vi "氨氮测量流程.vi"(10 "量程模式":T1, 11 "参数":T2={"站号"=1, "量程切换"=enum."AUTO", "控制命令"=enum."启动测量", "模式设置"=enum."待机", "测量间隔"=0} {"站号" items=["总磷"=1, "总氮"=2]}) -> ()   [LabVIEW 2016, in "氨氮.lvlib"]
uses:
  PLC/PLC.lvlib
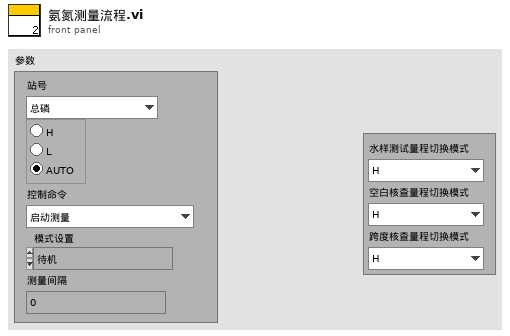
[diagram p1: front panel]
types:
  T1 = cluster{"水样测试量程切换模式":enum16{"H", "L", "AUTO"}, "空白核查量程切换模式":enum16{"H", "L", "AUTO"}, "跨度核查量程切换模式":enum16{"H", "L", "AUTO"}}
  T2 = cluster{"站号":u16, "量程切换":enum32{"H", "L", "AUTO"}, "控制命令":enum16{"启动测量", "标样核查", "零点核查", "跨度核查", "空白测试", "平行样测试", "加标回收", "空白校准", "标样校准", "初始化（清洗）", "停止测试", "仪器重启", "校时", "模式设置", "测量间隔设置"}, "模式设置":enum16{"待机", "连续模式", "周期模式", "定点模式", "受控模式", "手动模式"}, "测量间隔":u16}
  T3 = enum16{"初始化", "通电", "参数1启动", "等待参数1测试完成", "参数1测试完成", "参数1存储数据", "参数2启动", "等待参数2测试完成", "参数2测试完成", "参数2存储数据", "断电", "结束"}
  T4 = cluster{"时间标识":timestamp, "设备":string, "日志信息":string, "流程参数":string}
  T5 = cluster{"时间标识":timestamp, "监测值":sgl, "单位":u16, "数据标识":string, "因子编码":u32, "标样参考值":sgl, "F0":sgl, "F1":sgl, "F2":sgl, "F3":sgl, "温度":sgl, "湿度":sgl, "量程标识":string}
  T6 = enum16{"维护数据", "水样测试", "标样核查", "零点核查", "跨度核查", "空白测试", "平行样测试", "加标回收", "空白校准", "标样校准", "初始化（清洗）"}
  T7 = cluster{"系统时间":timestamp, "工作状态":enum16{"空闲", "水样测试", "标样核查", "零点核查", "跨度核查", "空白测试", "平行样测试", "加标回收", "空白校准", "标样校准", "初始化（清洗）"}, "测量模式":enum16{"待机", "连续模式", "周期模式", "定点模式", "受控模式", "手动模式"}, "告警代码":enum16{"无告警", "缺试剂告警", "缺水样告警", "缺蒸馏水告警", "缺标液告警", "仪表漏液告警", "标定异常告警", "超量程告警", "加热异常", "低试剂预警", "超上限告警", "超下限告警", "仪表内部其他异常", "滴定异常告警", "电极异常告警", "量程切换告警", "参数设置告警", "PH电极电位异常", "电导率电极异常", "浊度光度异常", "溶解氧电极异常", "溶解氧光强异常", "温度异常告警", "PH异常告警", "溶解氧异常告警", "电导率异常告警", "浊度异常告警", "叶绿素异常告警", "藻密度异常告警", "蓝绿藻异常告警", "ORP异常告警", "氨氮异常告警", "清洁刷异常告警", "SD卡异常告警", "蓝牙异常告警", "Wifi异常告警", "流程异常告警"}, "故障代码":enum16{"无故障", "电机故障", "温度故障", "通讯故障", "滴定故障"}, "日志代码":u16, "软件版本":u16, "F0":sgl, "F1":sgl, "F2":sgl, "F3":sgl, "T":sgl, "H":sgl, "id":u16, "flowid":u16, "量程":u16, "总磷控温温度1":sgl, "营养盐控温温度2":sgl, "ADC":sgl}
  T8 = enum16{"启动测量", "标样核查", "零点核查", "跨度核查", "空白测试", "平行样测试", "加标回收", "空白校准", "标样校准", "初始化（清洗）", "停止测试", "仪器重启", "校时", "模式设置", "测量间隔设置"}
  T9 = enum16{"空闲", "水样测试", "标样核查", "零点核查", "跨度核查", "空白测试", "平行样测试", "加标回收", "空白校准", "标样校准", "初始化（清洗）"}
  T10 = cluster{"跨度值":dbl, "零点标准液浓度":dbl, "跨度标准液浓度":dbl, "标准液标准浓度":dbl}
  T11 = cluster{"因子编码":u32, "单位":u16, "标样参考值":sgl, "水样数据时间":timestamp, "水样实测值":sgl, "水样数据标识":string, "标样数据时间":timestamp, "标样实测值":sgl, "标样数据标识":string, "空白数据时间":timestamp, "空白实测值":sgl, "空白数据标识":string, "零点核查数据时间":timestamp, "零点核查实测值":sgl, "零点核查数据标识":string, "跨度核查数据时间":timestamp, "跨度核查实测值":sgl, "跨度核查数据标识":string, "加标回收数据时间":timestamp, "加标回收实测值":sgl, "加标回收数据标识":string, "平行样数据时间":timestamp, "平行样实测值":sgl, "平行样数据标识":string}
  T12 = cluster{"运行模式":enum16{"维护模式", "常规模式", "应急模式", "质控模式"}}
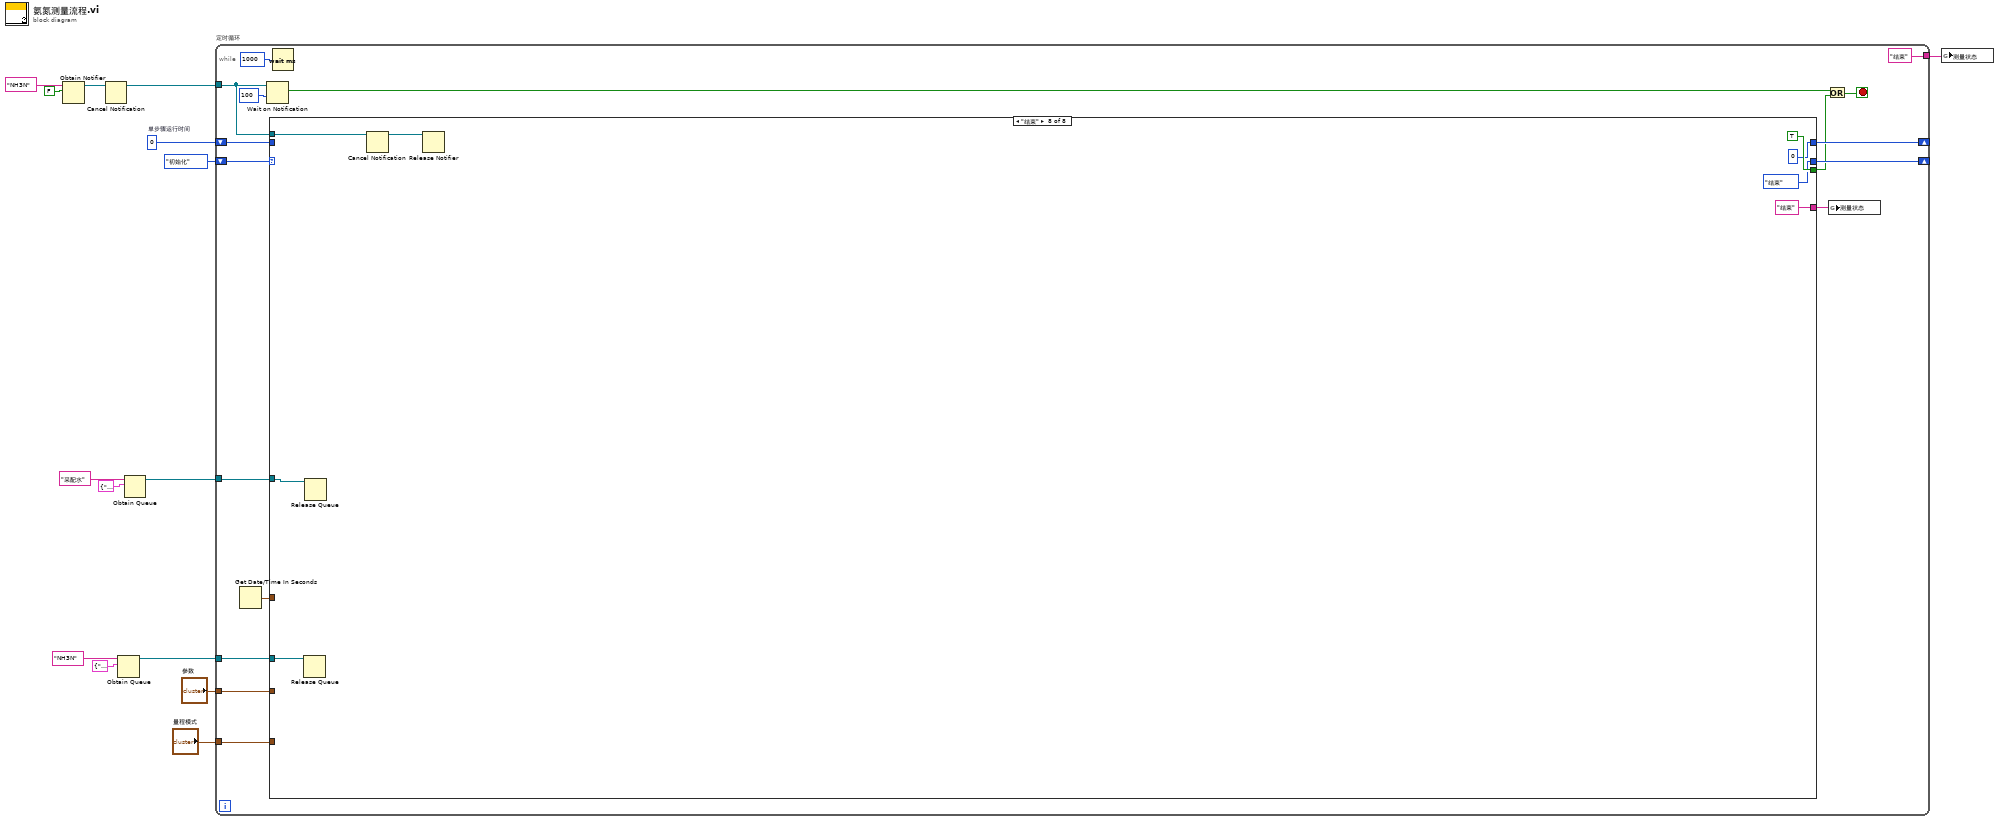
[diagram p0: block diagram]
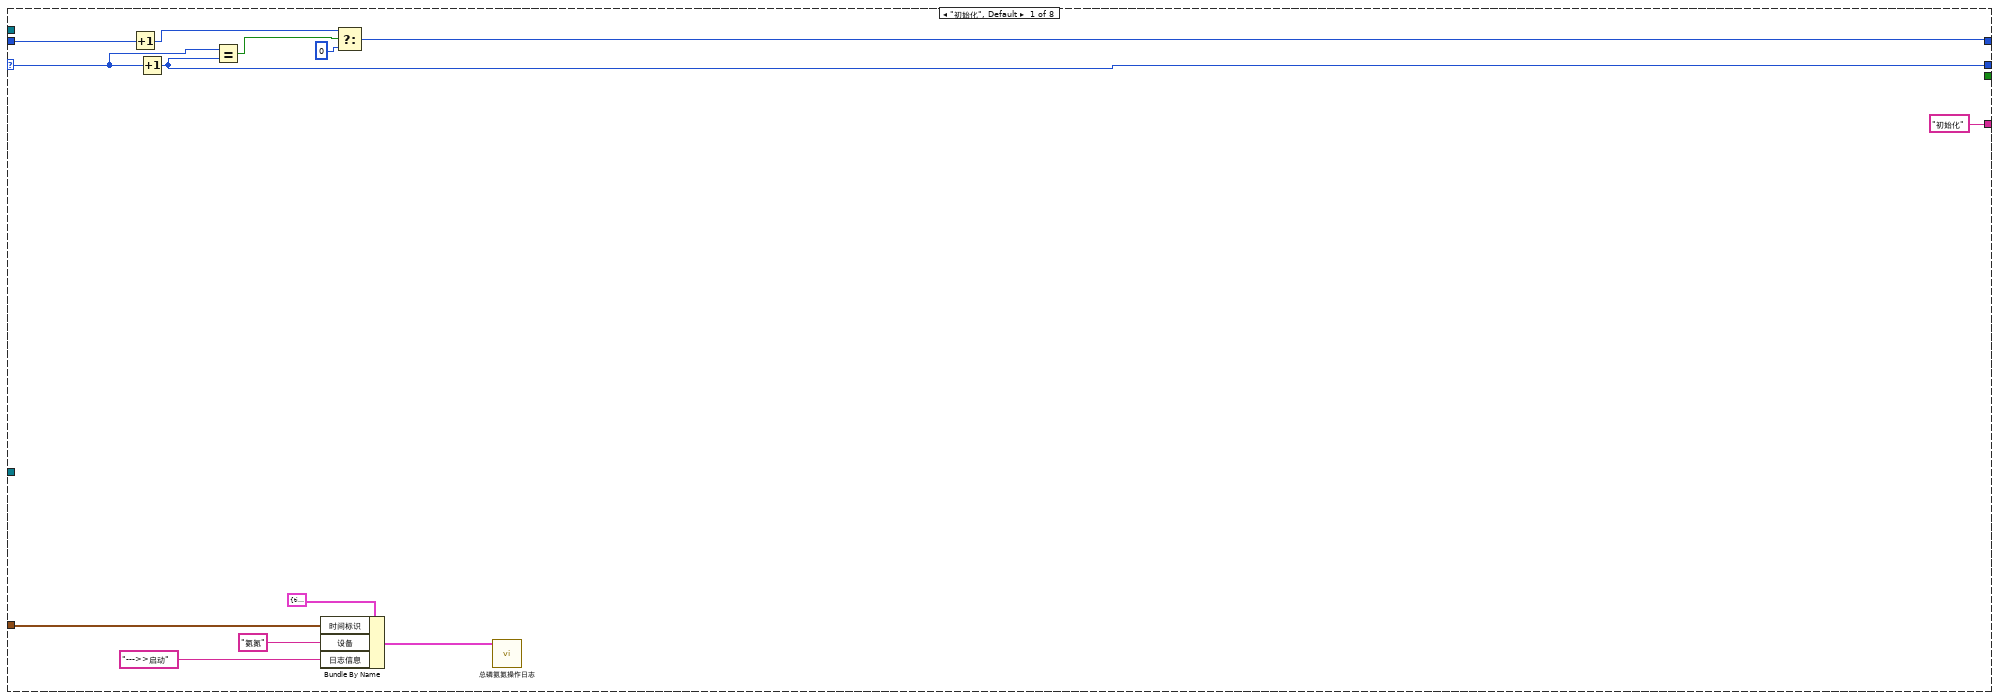
[diagram p2: hidden frame]
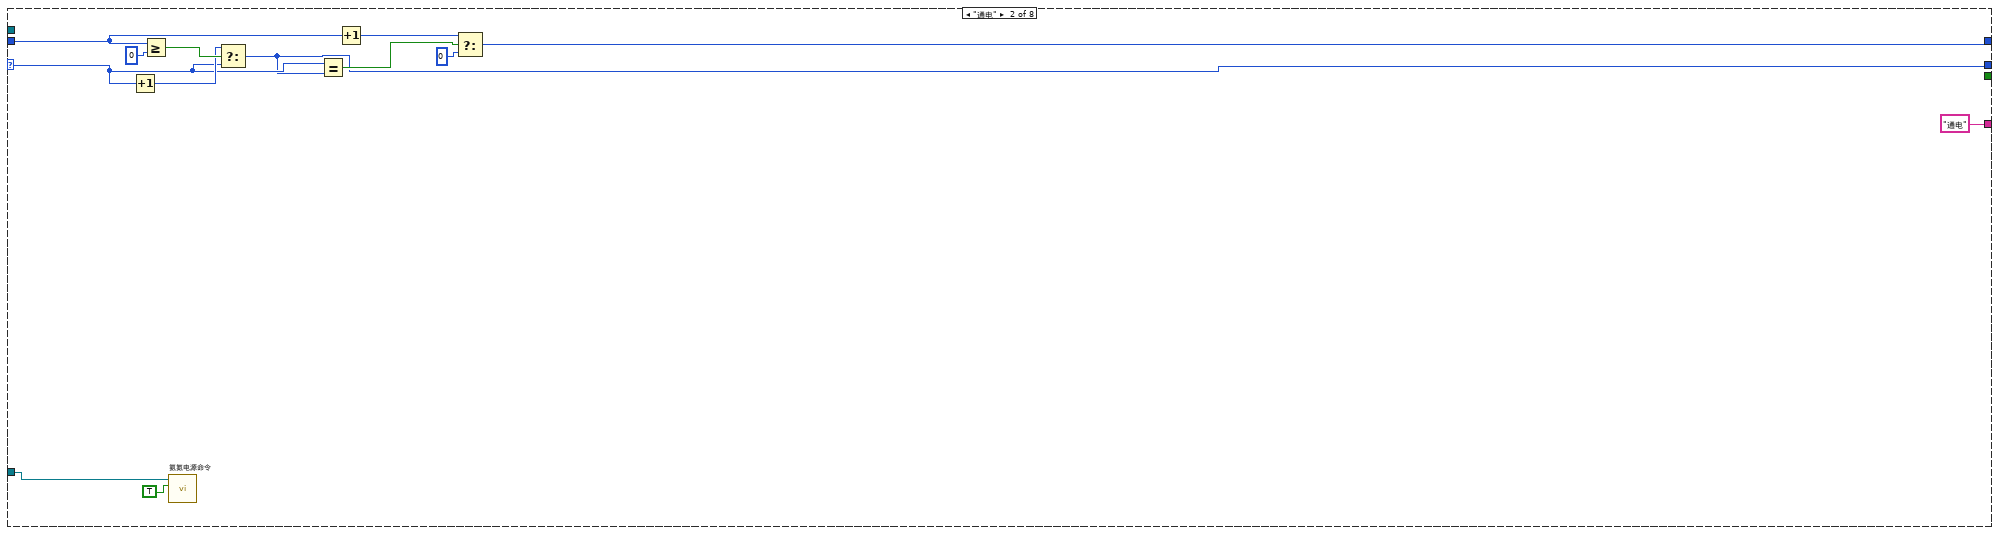
[diagram p3: hidden frame]
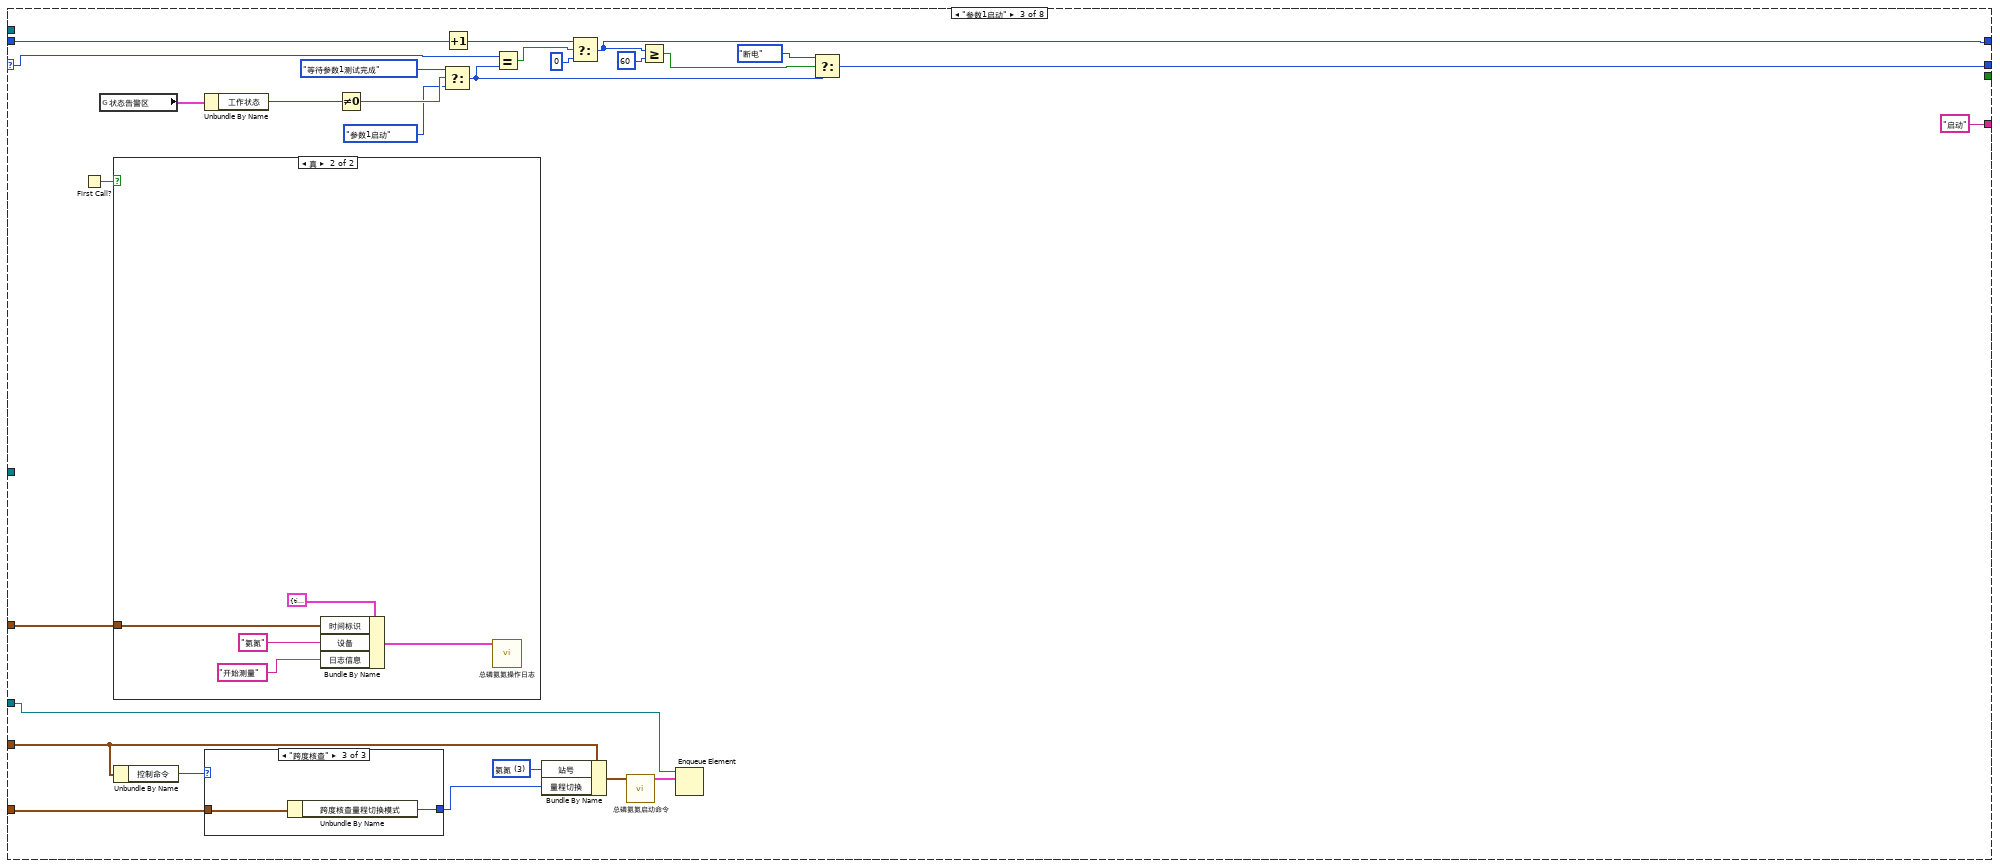
[diagram p4: hidden frame]
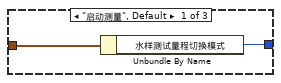
[diagram p5: hidden frame]
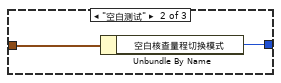
[diagram p6: hidden frame]
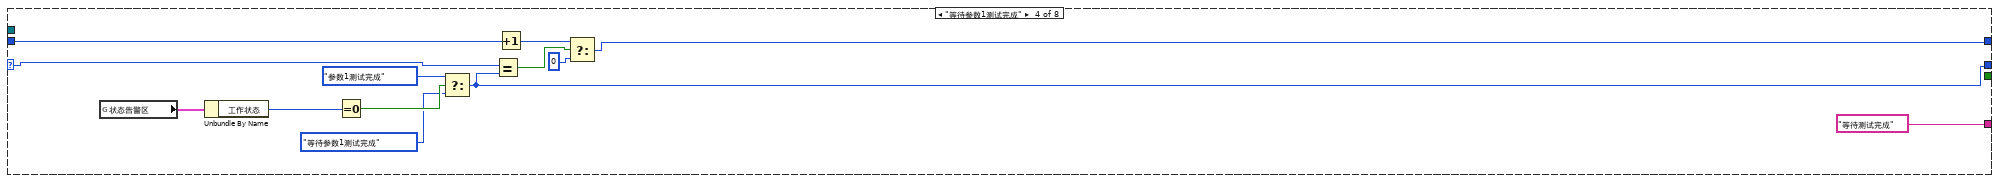
[diagram p8: hidden frame]
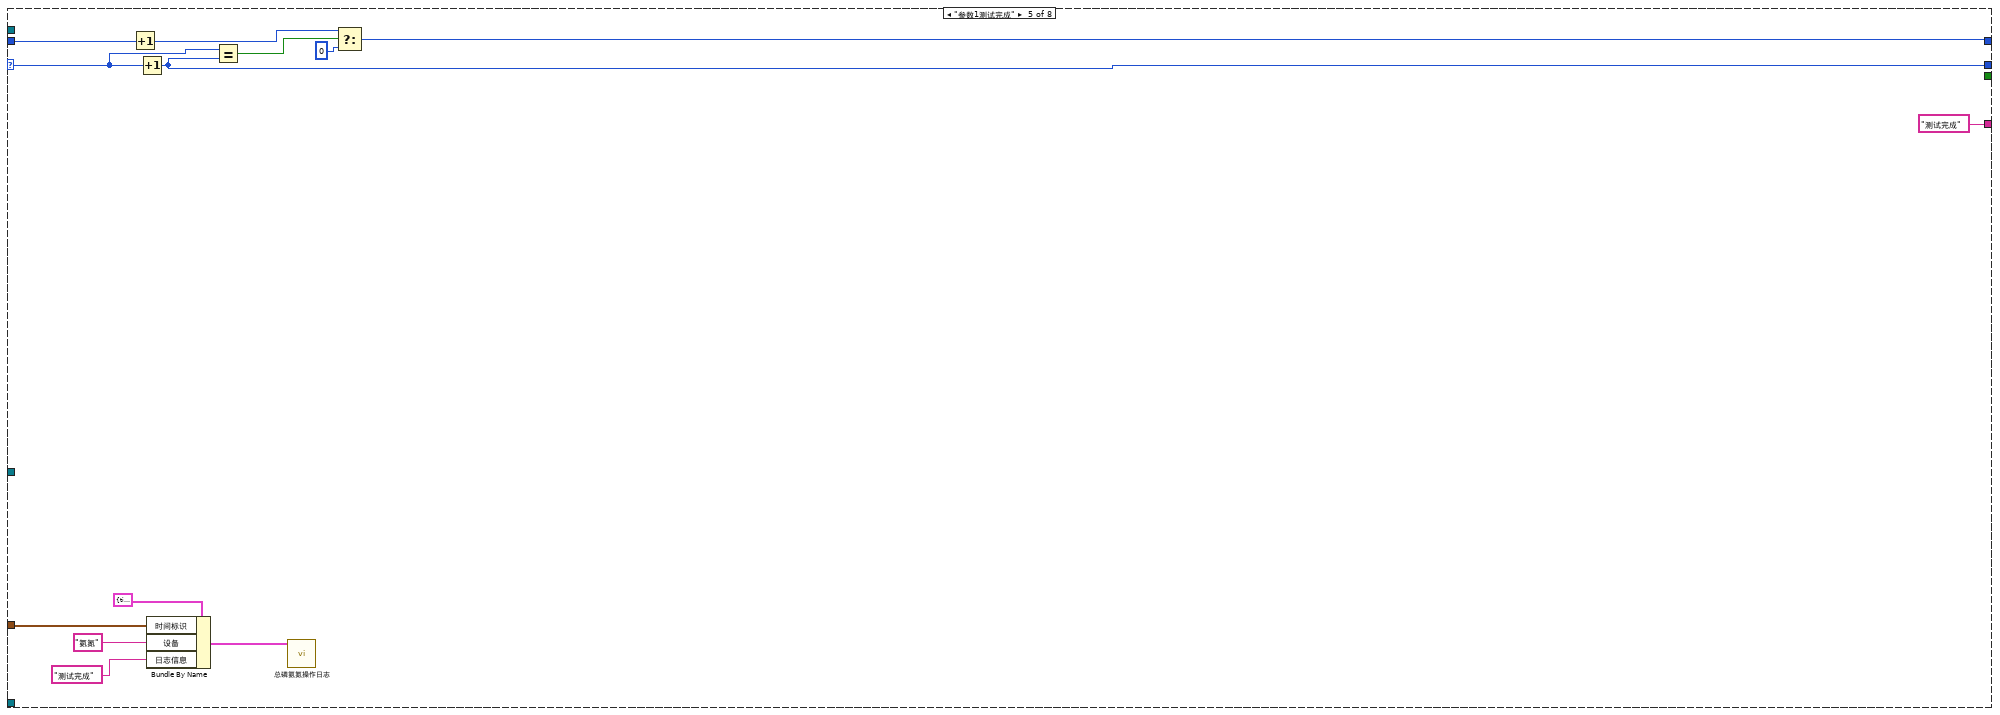
[diagram p9: hidden frame]
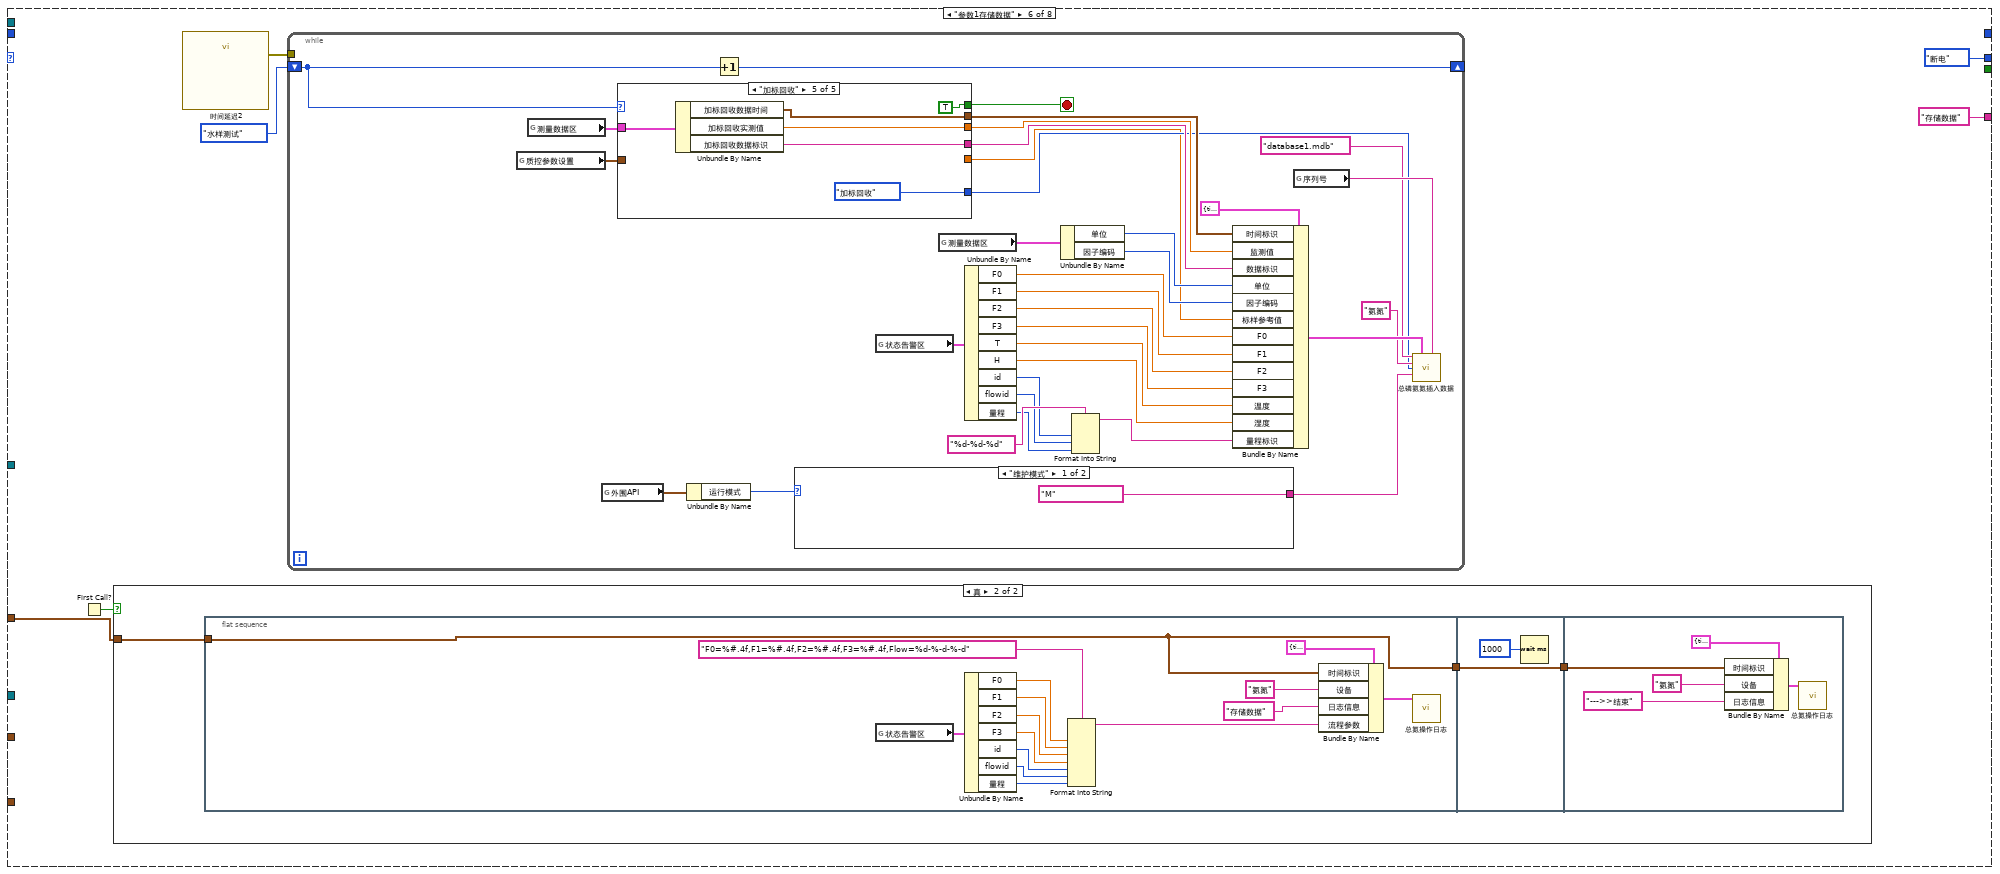
[diagram p10: hidden frame]
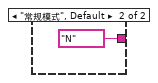
[diagram p11: hidden frame]
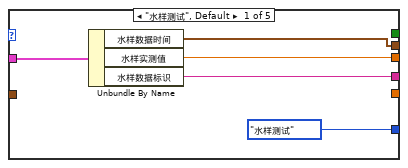
[diagram p12: hidden frame]
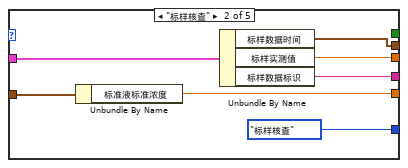
[diagram p13: hidden frame]
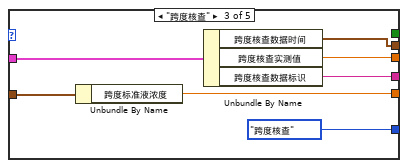
[diagram p14: hidden frame]
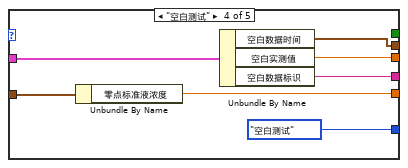
[diagram p15: hidden frame]
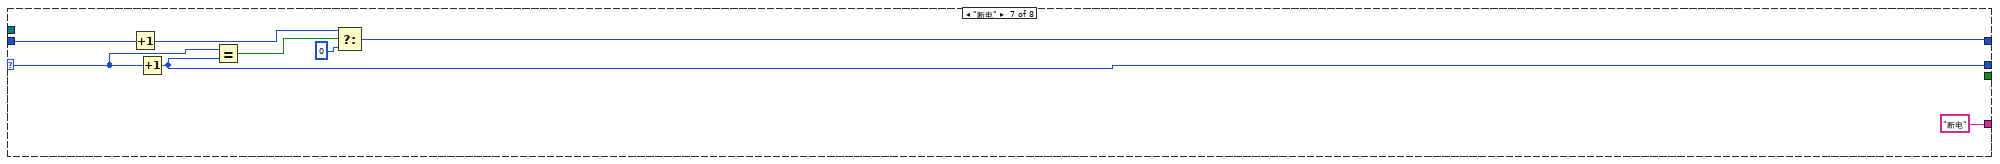
[diagram p17: hidden frame]
diagram:
  w11 = 0  # 单步骤运行时间
  n1 = Obtain Notifier(name (unnamed)="NH3N" ("名称（未命名）"), notification data type=FALSE) -> (notifier out=w8:refnum<notifier>)  [unwired: 2 in, 2 out]
  n2 = Cancel Notification(0:w8) -> (8:w7:refnum<notifier>)  [unwired: 1 in, 2 out]
  n3 = Obtain Queue(name (unnamed)="NH3N" ("名称（未命名）"), element data type=cluster{"命令":string, "data":variant} {"命令"="", "data"=variant}) -> (queue out=w12:refnum<queue>)  [unwired: 3 in, 2 out]
  n4 = Obtain Queue(name (unnamed)="采配水" ("名称（未命名）"), element data type=cluster{"命令":string, "数据":variant} {"命令"="", "数据"=variant}) -> (queue out=w1:refnum<queue>)  [unwired: 3 in, 2 out]
  n5 = while "定时循环" {
    shift-right: [w31] -> _
    shift-left: T3."初始化" ("枚举") -> [w32]
    tunnel: w12 -> [w30]
    shift-right: [w28] -> _
    shift-left: w11 -> [w29]
    tunnel: w7 -> [w27]
    tunnel: "参数" -> [w22]
    tunnel: "量程模式" -> [w19]
    tunnel: ["结束" ("输入 1")] -> w4
    tunnel: w1 -> [w16]
    stop <- w23 stop-if-true
    n6 = Get Date/Time In Seconds() -> (seconds since 1Jan1904=w20:timestamp)
    n7 = Wait on Notification(notifier=w27, timeout in ms (-1)=100 ("超时毫秒(-1)")) -> (notification=w24:bool)  [unwired: 2 in, 3 out]
    n8 = case shown="\"结束\"" w32 {
      selector: w32 -> [w43 w52 w80 w104 w119 _ w226 _]
      tunnel: [_ _ _ _ _ _ _ TRUE] -> w25
      tunnel: [w44 w51 w62 w103 w118 T3."断电" ("枚举") w225 T3."结束" ("枚举")] -> w31
      tunnel: w30 -> [_ _ w85 _ _ _ _ w234]
      tunnel: w29 -> [w45 w53 w81 w106 w120 _ w228 _]
      tunnel: [w41 w54 w67 w105 w121 _ w227 0 ("t")] -> w28
      tunnel: w27 -> [_ _ _ _ _ _ _ w233]
      tunnel: w22 -> [_ _ w71 _ _ _ _ _]
      tunnel: w20 -> [w35 _ w76 _ w112 w128 _ _]
      tunnel: ["初始化" ("输入 1") "通电" ("输入 1") "启动" ("输入 1") "等待测试完成" ("输入 1") "测试完成" ("输入 1") "存储数据" ("输入 1") "断电" ("输入 1") "结束" ("输入 1")] -> w18
      tunnel: w19 -> [_ _ w69 _ _ _ _ _]
      tunnel: w16 -> [_ w46 _ _ _ _ _ w229]
      frame "初始化", Default {
        n9 = Increment(x=w45) -> (x+1=w39:i32)
        n10 = Increment(x=w43) -> (x+1=w44:T3)
        n11 = Equal?(x=w43, y=w44) -> (x = y?=w42:bool)
        n12 = Bundle By Name(cluster=T4 {"时间标识"=timestamp(0 s since 1904-01-01), "设备"="", "日志信息"="", "流程参数"=""} ("data in"), "时间标识"=w35, "设备"="氨氮", "日志信息"="--->>启动") -> (w33:T4)
        n13 = Select(t=w39, s=w42, f=0 ("t")) -> (s? t:f=w41:i32)
        n14 = call "总磷氨氮操作日志.vi"("data in"=w33) -> ()  [unwired: 11 in]
      }
      frame "通电" {
        n15 = Increment(x=w52) -> (x+1=w56:T3)
        n16 = Greater Or Equal?(x=w53, y=0) -> (x >= y?=w57:bool)
        n17 = call "氨氮电源命令.vi"("通电/断电"=TRUE, "队列"=w46) -> ()  [unwired: 9 in, 1 out]
        n18 = Select(t=w56, s=w57, f=w52) -> (s? t:f=w51:T3)
        n19 = Equal?(x=w52, y=w51) -> (x = y?=w55:bool)
        n20 = Increment(x=w53) -> (x+1=w50:i32)
        n21 = Select(t=w50, s=w55, f=0 ("t")) -> (s? t:f=w54:i32)
      }
      frame "参数1启动" {
        w77 = u16 3 items=["总磷"=1, "总氮"=2, "氨氮"=3] ("站号")
        n22 = First Call?() -> (First Call?: T/F=w75:bool)
        n23 = global read "VAR总磷氨氮全局变量.vi" "状态告警区"() -> (w59:T7)
        n24 = case shown="真" w75 {
          tunnel: w76 -> [_ w93]
          frame False {
          }
          frame True {
            n25 = Bundle By Name(cluster=T4 {"时间标识"=timestamp(0 s since 1904-01-01), "设备"="", "日志信息"="", "流程参数"=""} ("data in"), "时间标识"=w93, "设备"="氨氮", "日志信息"="开始测量") -> (w92:T4)
            n26 = call "总磷氨氮操作日志.vi"("data in"=w92) -> ()  [unwired: 11 in]
          }
        }
        n27 = Unbundle By Name(w71) -> ("控制命令"=w70:T8)
        n28 = Unbundle By Name(w59) -> ("工作状态"=w84:T9)
        n29 = case shown="\"跨度核查\"" w70 {
          tunnel: w69 -> [w87 w89 w91]
          tunnel: [w86 w88 w90] -> w68
          frame "启动测量", Default {
            n30 = Unbundle By Name(w87) -> ("水样测试量程切换模式"=w86:enum16{"H", "L", "AUTO"})
          }
          frame "空白测试" {
            n31 = Unbundle By Name(w89) -> ("空白核查量程切换模式"=w88:enum16{"H", "L", "AUTO"})
          }
          frame "跨度核查" {
            n32 = Unbundle By Name(w91) -> ("跨度核查量程切换模式"=w90:enum16{"H", "L", "AUTO"})
          }
        }
        n33 = Not Equal To 0?(x=w84) -> (x != 0?=w83:bool)
        n34 = Select(t=T3."等待参数1测试完成" ("枚举"), s=w83, f=T3."参数1启动" ("枚举")) -> (s? t:f=w64:T3)
        n35 = Increment(x=w81) -> (x+1=w78:i32)
        n36 = Equal?(x=w80, y=w64) -> (x = y?=w82:bool)
        n37 = Bundle By Name(cluster=w71, "站号"=w77, "量程切换"=w68) -> (w61:T2)
        n38 = Select(t=w78, s=w82, f=0 ("t")) -> (s? t:f=w67:i32)
        n39 = call "总磷氨氮启动命令.vi"("参数"=w61) -> ("启动命令"=w60:cluster{"命令":string, "data":variant})  [unwired: 10 in]
        n40 = Greater Or Equal?(x=w67, y=60) -> (x >= y?=w65:bool)
        n41 = Enqueue Element(queue=w85, element=w60) -> ()  [unwired: 2 in, 3 out]
        n42 = Select(t=T3."断电" ("枚举"), s=w65, f=w64) -> (s? t:f=w62:T3)
      }
      frame "等待参数1测试完成" {
        n43 = global read "VAR总磷氨氮全局变量.vi" "状态告警区"() -> (w97:T7)
        n44 = Unbundle By Name(w97) -> ("工作状态"=w109:T9)
        n45 = Equal To 0?(x=w109) -> (x = 0?=w108:bool)
        n46 = Select(t=T3."参数1测试完成" ("枚举"), s=w108, f=T3."等待参数1测试完成" ("枚举")) -> (s? t:f=w103:T3)
        n47 = Equal?(x=w104, y=w103) -> (x = y?=w107:bool)
        n48 = Increment(x=w106) -> (x+1=w101:i32)
        n49 = Select(t=w101, s=w107, f=0 ("t")) -> (s? t:f=w105:i32)
      }
      frame "参数1测试完成" {
        n50 = Increment(x=w120) -> (x+1=w116:i32)
        n51 = Increment(x=w119) -> (x+1=w118:T3)
        n52 = Bundle By Name(cluster=T4 {"时间标识"=timestamp(0 s since 1904-01-01), "设备"="", "日志信息"="", "流程参数"=""} ("data in"), "时间标识"=w112, "设备"="氨氮", "日志信息"="测试完成") -> (w110:T4)
        n53 = Equal?(x=w119, y=w118) -> (x = y?=w122:bool)
        n54 = call "总磷氨氮操作日志.vi"("data in"=w110) -> ()  [unwired: 11 in]
        n55 = Select(t=w116, s=w122, f=0 ("t")) -> (s? t:f=w121:i32)
      }
      frame "参数1存储数据" {
        n56 = First Call?() -> (First Call?: T/F=w126:bool)
        n57 = case shown="真" w126 {
          tunnel: w128 -> [_ w198]
          frame False {
          }
          frame True {
            n58 = flat-sequence {
              tunnel: w198 -> [w210]
              tunnel: [w210] -> w197
              tunnel: w197 -> [w215]
              tunnel: [w215] -> w196
              tunnel: w196 -> [w217]
              frame #0 {
                n59 = global read "VAR总磷氨氮全局变量.vi" "状态告警区"() -> (w200:T7)
                n60 = Unbundle By Name(w200) -> ("F0"=w202:sgl, "F1"=w203:sgl, "F2"=w204:sgl, "F3"=w205:sgl, "id"=w206:u16, "flowid"=w207:u16, "量程"=w208:u16)
                n61 = Format Into String(format string="F0=%#.4f,F1=%#.4f,F2=%#.4f,F3=%#.4f,Flow=%d-%-d-%-d" ("格式字符串"), w202, w203, w204, w205, w206, w207, w208) -> (resulting string=w201:string)  [unwired: 2 in, 1 out]
                n62 = Bundle By Name(cluster=T4 {"时间标识"=timestamp(0 s since 1904-01-01), "设备"="", "日志信息"="", "流程参数"=""} ("data in"), "时间标识"=w210, "设备"="氨氮", "日志信息"="存储数据", "流程参数"=w201) -> (w199:T4)
                n63 = call "总氮操作日志.vi"("data in"=w199) -> ()  [unwired: 11 in]
              }
              frame #1 {
                n64 = Wait (ms)(milliseconds to wait=u32 1000 ("等待时间（毫秒）")) -> ()  [unwired: 1 out]
              }
              frame #2 {
                n65 = Bundle By Name(cluster=T4 {"时间标识"=timestamp(0 s since 1904-01-01), "设备"="", "日志信息"="", "流程参数"=""} ("data in"), "时间标识"=w217, "设备"="氨氮", "日志信息"="--->>结束") -> (w216:T4)
                n66 = call "总氮操作日志.vi"("data in"=w216) -> ()  [unwired: 11 in]
              }
            }
          }
        }
        n67 = call "时间延迟2"() -> ("error out"=w123:errorcluster)  [unwired: 11 in]
        n68 = while {
          shift-right: [w155] -> _
          shift-left: enum16{"水样测试", "标样核查", "跨度核查", "空白测试", "加标回收"}."水样测试" ("测量模式") -> [w156]
          tunnel: w123 -> [_]
          stop <- w157 stop-if-true
          n69 = global read "氨氮断电保存全局变量.vi" "质控参数设置"() -> (w130:T10)
          n70 = global read "VAR总磷氨氮全局变量.vi" "测量数据区"() -> (w149:T11)
          n71 = global read "VAR总磷氨氮全局变量.vi" "外围API"() -> (w133:T12)
          n72 = case shown="\"加标回收\"" w156 {
            tunnel: w149 -> [w164 w171 w178 w185 w190]
            tunnel: [w168 w175 w182 w189 w195] -> w154
            tunnel: [w167 w174 w181 w188 w194] -> w153
            tunnel: [w166 w173 w180 w187 w193] -> w152
            tunnel: [T6."水样测试" ("测量模式") T6."标样核查" ("测量模式") T6."跨度核查" ("测量模式") T6."空白测试" ("测量模式") T6."加标回收" ("测量模式")] -> w141
            tunnel: [_ _ _ _ TRUE] -> w157
            tunnel: w130 -> [_ w170 w177 w184 _]
            tunnel: [_ w169 w176 w183 _] -> w129
            frame "水样测试", Default {
              n73 = Unbundle By Name(w164) -> ("水样数据时间"=w168:timestamp, "水样实测值"=w167:sgl, "水样数据标识"=w166:string)
            }
            frame "标样核查" {
              n74 = Unbundle By Name(w170) -> ("标准液标准浓度"=w169:dbl)
              n75 = Unbundle By Name(w171) -> ("标样数据时间"=w175:timestamp, "标样实测值"=w174:sgl, "标样数据标识"=w173:string)
            }
            frame "跨度核查" {
              n76 = Unbundle By Name(w177) -> ("跨度标准液浓度"=w176:dbl)
              n77 = Unbundle By Name(w178) -> ("跨度核查数据时间"=w182:timestamp, "跨度核查实测值"=w181:sgl, "跨度核查数据标识"=w180:string)
            }
            frame "空白测试" {
              n78 = Unbundle By Name(w184) -> ("零点标准液浓度"=w183:dbl)
              n79 = Unbundle By Name(w185) -> ("空白数据时间"=w189:timestamp, "空白实测值"=w188:sgl, "空白数据标识"=w187:string)
            }
            frame "加标回收" {
              n80 = Unbundle By Name(w190) -> ("加标回收数据时间"=w195:timestamp, "加标回收实测值"=w194:sgl, "加标回收数据标识"=w193:string)
            }
          }
          n81 = Unbundle By Name(w133) -> ("运行模式"=w132:enum16{"维护模式", "常规模式", "应急模式", "质控模式"})
          n82 = Increment(x=w156) -> (x+1=w155:enum16{"水样测试", "标样核查", "跨度核查", "空白测试", "加标回收"})
          n83 = case shown="\"维护模式\"" w132 {
            tunnel: ["M" ("数据标记表") "N" ("数据标记表")] -> w131
            frame "维护模式" {
            }
            frame "常规模式", Default {
            }
          }
          n84 = global read "VAR总磷氨氮全局变量.vi" "状态告警区"() -> (w147:T7)
          n85 = global read "VAR总磷氨氮全局变量.vi" "测量数据区"() -> (w148:T11)
          n86 = Unbundle By Name(w147) -> ("F0"=w139:sgl, "F1"=w138:sgl, "F2"=w137:sgl, "F3"=w136:sgl, "T"=w135:sgl, "H"=w134:sgl, "id"=w160:u16, "flowid"=w159:u16, "量程"=w158:u16)
          n87 = Unbundle By Name(w148) -> ("单位"=w151:u16, "因子编码"=w150:u32)
          n88 = Format Into String(format string="%d-%d-%d" ("格式字符串"), w160, w159, w158) -> (resulting string=w140:string)  [unwired: 2 in, 1 out]
          n89 = Bundle By Name(cluster=T5 {"时间标识"=timestamp(0 s since 1904-01-01), "监测值"=0.0, "单位"=0, "数据标识"="", "因子编码"=0, "标样参考值"=0.0, "F0"=0.0, "F1"=0.0, "F2"=0.0, "F3"=0.0, "温度"=0.0, "湿度"=0.0, "量程标识"=""} ("data"), "时间标识"=w154, "监测值"=w153, "数据标识"=w152, "单位"=w151, "因子编码"=w150, "标样参考值"=w129, "F0"=w139, "F1"=w138, "F2"=w137, "F3"=w136, "温度"=w135, "湿度"=w134, "量程标识"=w140) -> (w145:T5)
          n90 = global read "VAR总磷氨氮全局变量.vi" "序列号"() -> (w144:string)
          n91 = call "总磷氨氮插入数据.vi"("database"="database1.mdb", "data"=w145, "SN"=w144, "table"="氨氮", "测量模式"=w141, "数据标记表"=w131) -> ()  [unwired: 9 in, 1 out]
        }
      }
      frame "断电" {
        n92 = Increment(x=w228) -> (x+1=w221:i32)
        n93 = Increment(x=w226) -> (x+1=w225:T3)
        n94 = Equal?(x=w226, y=w225) -> (x = y?=w223:bool)
        n95 = Select(t=w221, s=w223, f=0 ("t")) -> (s? t:f=w227:i32)
      }
      frame "结束" {
        n96 = Release Queue(queue=w234) -> ()  [unwired: 2 in, 3 out]
        n97 = Release Queue(queue=w229) -> ()  [unwired: 2 in, 3 out]
        n98 = Cancel Notification(0:w233) -> (8:w232:refnum<notifier>)  [unwired: 1 in, 2 out]
        n99 = Release Notifier(notifier=w232) -> ()  [unwired: 2 in, 3 out]
      }
    }
    n100 = Wait (ms)(milliseconds to wait=u32 1000 ("等待时间（毫秒）")) -> ()  [unwired: 1 out]
    n101 = Or(x=w24, y=w25) -> (x .or. y?=w23:bool)
    n102 = global write "VAR总磷氨氮全局变量.vi" "测量状态"(w18) -> ()
  }
  n103 = global write "VAR总磷氨氮全局变量.vi" "测量状态"(w4) -> ()
